vi "SetIntermediateCalibration3.vi"(8 "error in (no error)":errorcluster, 10 "Calibration table":T1={"version"=3, "table type"=60479, "table size"=496, "full version"=67109888, "crc32"=3963612841, "baseline"=-54.831806, "model"=1, "fx left"=917.7658, "fy left"=915.4345, "px left"=631.39185, "py left"=376.6227, "py right"=364.3492, "px right"=651.2822, "fy right"=921.49005, "fx right"=923.5849, "k left"=[0.13533829, -0.40519878, 0.0008784002, -0.0011180333, 0.3588802], "k right"=[0.12740475, -0.39763576, 0.00037952562, -0.0022863527, 0.35284942], "RLeft"=[0.9999986, 0.0009555143, -0.001359244, -0.0009574645, 0.9999985, -0.001434832, 0.001357871, 0.0014361315, 0.99999803], "Rright"=[0.99998456, -0.0019937593, -0.0051888847, 0.002001206, 0.99999696, 0.0014302958, 0.0051860176, -0.0014406577, 0.9999855], "uint8 reserved1"=[0, 0, 0, 0, 0, 0, 0, 0, 0, 0, 0, 0, 0, 0, 0, 0, 0, 0, 0, 0, 0, 0, 0, 0, 0, 0, 0, 0, 0, 0, 0, 0, 0, 0, 0, 0, 0, 0, 0, 0, 0, 0, 0, 0, 0, 0, 0, 0, 0, 0, 0, 0, 0, 0, 0, 0, 0, 0, 0, 0, 0, 0, 0, 0, 0, 0, 0, 0, 0, 0, 0, 0, 0, 0, 0, 0, 0, 0, 0, 0, 0, 0, 0, 0, 0, 0, 0, 0], "uint8 reserved2"=[0, 0, 0, 0, 0, 0, 0, 0, 0, 0, 0, 0, 0, 0, 0, 0, 0, 0, 0, 0, 0, 0, 0, 0, 0, 0, 0, 0, 0, 0, 0, 0, 0, 0, 0, 0, 0, 0, 0, 0, 0, 0, 0, 0, 0, 0, 0, 0, 0, 0, 0, 0, 0, 0, 0, 0, 0, 0, 0, 0, 0, 0, 0, 0], "1920x1080"=[1428.9095, 1428.9095, 951.85925, 556.0496], "1280x720"=[952.6064, 952.6064, 634.5728, 370.69974], "640x480"=[635.0709, 635.0709, 316.38187, 247.13316], "848x480"=[635.0709, 635.0709, 420.38187, 247.13316], "640x360"=[476.3032, 476.3032, 317.2864, 185.34987], "424x240"=[317.53546, 317.53546, 210.19093, 123.56658], "320x240"=[317.53546, 317.53546, 158.19093, 123.56658], "480x270"=[357.2274, 357.2274, 237.96481, 139.0124], "1280x800"=[1058.4515, 1058.4515, 633.9698, 411.8886], "960x540"=[714.4548, 714.4548, 475.92963, 278.0248], "Reserved1"=[714.4548, 714.4548, 475.92963, 278.0248], "Reserved 2"=[714.4548, 714.4548, 475.92963, 278.0248]} {"crc32" format="%x"}, 11 "Input Calibration Parameters":T3={"fx"=0.7094939, "fy"=1.2617997, "px"=0.49358395, "py"=0.4803248, "k left"=[0.13808699, -0.41154006, 0.00043059044, 0.00047021545, 0.34858656], "fx2"=0.7124277, "fy2"=1.2668592, "py2"=0.4684578, "px2"=0.4979801, "k right"=[0.14090613, -0.42654052, -0.0003404384, 0.0005577445, 0.36482877], "RLeft"=[0.99998826, -0.004810224, 0.0006247892, 0.0048055355, 0.9999618, 0.0073000034, -0.00065988, -0.007296915, 0.9999732], "Rright"=[0.9999898, 0.00018351649, -0.0045086313, -0.00021641784, 0.99997336, -0.0072980113, 0.004507172, 0.007298913, 0.9999632], "baseline"=-55.153587, "useBrownModel"=1, "1280x720"=[961.38745, 961.38745, 632.941, 342.07367]}) -> (0 "error out":errorcluster, 2 "size(s)":i32=256, 3 "Intermediate Output":u8[](array[numeric])=[156, 141, 55, 63, 113, 190, 162, 63, 62, 252, 142, 135, 63, 5, 233, 9, 31, 150, 10, 62, 55, 118, 207, 190, 113, 68, 102, 58, 249, 138, 146, 186, 37, 191, 183, 62, 140, 183, 56, 63, 9, 210, 163, 63, 224, 139, 1, 63, 166, 65, 2, 63, 100, 118, 2, 62, 234, 150, 203, 190, 17, 251, 198, 57, 162, 214, 21, 187, 174, 168, 180, 62, 233, 255, 127, 63, 123, 123, 122, 58, 169, 40, 178, 186, 91, 254, 122, 186, 231, 255, 127, 63, 249, 16, 188, 186, 151, 250, 177, 58, 148, 60, 188, 58, 223, 255, 127, 63, 253, 254, 127, 63, 187, 169, 2, 187, 133, 7, 170, 187, 170, 38, 3, 59, 205, 255, 127, 63, 195, 120, 187, 58, 120, 239, 169, 59, 115, 212, 188, 186, 13, 255, 127, 63, 197, 83, 91, 194, 1, 0, 0, 0, 0, 0, 0, 0, 0, 0, 0, 0, 0, 0, 0, 0, 0, 0, 0, 0, 0, 0, 0, 0, 0, 0, 0, 0, 0, 0, 0, 0, 0, 0, 0, 0, 0, 0, 0, 0, 0, 0, 0, 0, 0, 0, 0, 0, 0, 0, 0, 0, 0, 0, 0, 0, 0, 0, 0, 0, 0, 0, 0, 0, 0, 0, 0, 0, 0, 0, 0, 0, 0, 0, 0, 0, 0, 0, 0, 0, 0, 0, 0, 0, 0, 0, 0, 0, 0, 0, 0, 0, 207, 38, 110, 68, 207, 38, 110, 68, 169, 164, 30, 68, 145, 89, 185, 67] format="%x", 4 "New Full cal. output":u8[](array[numeric])=[3, 0, 25, 0, 240, 1, 0, 0, 0, 4, 0, 4, 169, 238, 63, 236, 156, 141, 55, 63, 113, 190, 162, 63, 135, 142, 252, 62, 9, 233, 5, 63, 31, 150, 10, 62, 55, 118, 207, 190, 113, 68, 102, 58, 249, 138, 146, 186, 37, 191, 183, 62, 140, 183, 56, 63, 9, 210, 163, 63, 166, 65, 2, 63, 224, 139, 1, 63, 100, 118, 2, 62, 234, 150, 203, 190, 17, 251, 198, 57, 162, 214, 21, 187, 174, 168, 180, 62, 233, 255, 127, 63, 123, 123, 122, 58, 169, 40, 178, 186, 91, 254, 122, 186, 231, 255, 127, 63, 249, 16, 188, 186, 151, 250, 177, 58, 148, 60, 188, 58, 223, 255, 127, 63, 253, 254, 127, 63, 187, 169, 2, 187, 133, 7, 170, 187, 170, 38, 3, 59, 205, 255, 127, 63, 195, 120, 187, 58, 120, 239, 169, 59, 115, 212, 188, 186, 13, 255, 127, 63, 197, 83, 91, 194, 1, 0, 0, 0, 0, 0, 0, 0, 0, 0, 0, 0, 0, 0, 0, 0, 0, 0, 0, 0, 0, 0, 0, 0, 0, 0, 0, 0, 0, 0, 0, 0, 0, 0, 0, 0, 0, 0, 0, 0, 0, 0, 0, 0, 0, 0, 0, 0, 0, 0, 0, 0, 0, 0, 0, 0, 0, 0, 0, 0, 0, 0, 0, 0, 0, 0, 0, 0, 0, 0, 0, 0, 0, 0, 0, 0, 0, 0, 0, 0, 0, 0, 0, 0, 0, 0, 0, 0, 0, 0, 0, 0, 27, 157, 178, 68, 27, 157, 178, 68, 254, 246, 109, 68, 45, 3, 11, 68, 207, 38, 110, 68, 207, 38, 110, 68, 169, 164, 30, 68, 145, 89, 185, 67, 138, 196, 30, 68, 138, 196, 30, 68, 225, 48, 158, 67, 23, 34, 119, 67, 138, 196, 30, 68, 138, 196, 30, 68, 225, 48, 210, 67, 23, 34, 119, 67, 207, 38, 238, 67, 207, 38, 238, 67, 169, 164, 158, 67, 145, 89, 57, 67, 138, 196, 158, 67, 138, 196, 158, 67, 225, 48, 82, 67, 23, 34, 247, 66, 138, 196, 158, 67, 138, 196, 158, 67, 225, 48, 30, 67, 23, 34, 247, 66, 27, 157, 178, 67, 27, 157, 178, 67, 254, 246, 109, 67, 45, 3, 11, 67, 115, 78, 132, 68, 115, 78, 132, 68, 17, 126, 30, 68, 190, 241, 205, 67, 27, 157, 50, 68, 27, 157, 50, 68, 254, 246, 237, 67, 45, 3, 139, 67, 0, 0, 0, 0, 0, 0, 0, 0, 0, 0, 0, 0, 0, 0, 0, 0, 0, 0, 0, 0, 0, 0, 0, 0, 0, 0, 0, 0, 0, 0, 0, 0, 0, 0, 0, 0, 0, 0, 0, 0, 0, 0, 0, 0, 0, 0, 0, 0, 0, 0, 0, 0, 0, 0, 0, 0, 0, 0, 0, 0, 0, 0, 0, 0, 0, 0, 0, 0, 0, 0, 0, 0, 0, 0, 0, 0, 0, 0, 0, 0, 0, 0, 0, 0, 0, 0, 0, 0, 0, 0, 0, 0, 0, 0, 0, 0] format="%x", 5 "New Calibration table":T1={"version"=3, "table type"=60479, "table size"=496, "full version"=67109888, "crc32"=3963612841, "baseline"=-54.831806, "model"=1, "fx left"=917.7658, "fy left"=915.4345, "px left"=631.39185, "py left"=376.6227, "py right"=364.3492, "px right"=651.2822, "fy right"=921.49005, "fx right"=923.5849, "k left"=[0.13533829, -0.40519878, 0.0008784002, -0.0011180333, 0.3588802], "k right"=[0.12740475, -0.39763576, 0.00037952562, -0.0022863527, 0.35284942], "RLeft"=[0.9999986, 0.0009555143, -0.001359244, -0.0009574645, 0.9999985, -0.001434832, 0.001357871, 0.0014361315, 0.99999803], "Rright"=[0.99998456, -0.0019937593, -0.0051888847, 0.002001206, 0.99999696, 0.0014302958, 0.0051860176, -0.0014406577, 0.9999855], "uint8 reserved1"=[0, 0, 0, 0, 0, 0, 0, 0, 0, 0, 0, 0, 0, 0, 0, 0, 0, 0, 0, 0, 0, 0, 0, 0, 0, 0, 0, 0, 0, 0, 0, 0, 0, 0, 0, 0, 0, 0, 0, 0, 0, 0, 0, 0, 0, 0, 0, 0, 0, 0, 0, 0, 0, 0, 0, 0, 0, 0, 0, 0, 0, 0, 0, 0, 0, 0, 0, 0, 0, 0, 0, 0, 0, 0, 0, 0, 0, 0, 0, 0, 0, 0, 0, 0, 0, 0, 0, 0], "uint8 reserved2"=[0, 0, 0, 0, 0, 0, 0, 0, 0, 0, 0, 0, 0, 0, 0, 0, 0, 0, 0, 0, 0, 0, 0, 0, 0, 0, 0, 0, 0, 0, 0, 0, 0, 0, 0, 0, 0, 0, 0, 0, 0, 0, 0, 0, 0, 0, 0, 0, 0, 0, 0, 0, 0, 0, 0, 0, 0, 0, 0, 0, 0, 0, 0, 0], "1920x1080"=[1428.9095, 1428.9095, 951.85925, 556.0496], "1280x720"=[952.6064, 952.6064, 634.5728, 370.69974], "640x480"=[635.0709, 635.0709, 316.38187, 247.13316], "848x480"=[635.0709, 635.0709, 420.38187, 247.13316], "640x360"=[476.3032, 476.3032, 317.2864, 185.34987], "424x240"=[317.53546, 317.53546, 210.19093, 123.56658], "320x240"=[317.53546, 317.53546, 158.19093, 123.56658], "480x270"=[357.2274, 357.2274, 237.96481, 139.0124], "1280x800"=[1058.4515, 1058.4515, 633.9698, 411.8886], "960x540"=[714.4548, 714.4548, 475.92963, 278.0248], "Reserved1"=[714.4548, 714.4548, 475.92963, 278.0248], "Reserved 2"=[714.4548, 714.4548, 475.92963, 278.0248]} {"crc32" format="%x"}, 6 "New size full":i32=512)   [LabVIEW 2017, in "libRealSense3.lvlib"]
uses:
  libRealSense3.lvlib
panel:
  in  "Calibration table 2":T1={"version"=3, "table type"=60479, "table size"=496, "full version"=67109888, "crc32"=3963612841, "baseline"=-54.831806, "model"=1, "fx left"=917.7658, "fy left"=915.4345, "px left"=631.39185, "py left"=376.6227, "py right"=364.3492, "px right"=651.2822, "fy right"=921.49005, "fx right"=923.5849, "k left"=[0.13533829, -0.40519878, 0.0008784002, -0.0011180333, 0.3588802], "k right"=[0.12740475, -0.39763576, 0.00037952562, -0.0022863527, 0.35284942], "RLeft"=[0.9999986, 0.0009555143, -0.001359244, -0.0009574645, 0.9999985, -0.001434832, 0.001357871, 0.0014361315, 0.99999803], "Rright"=[0.99998456, -0.0019937593, -0.0051888847, 0.002001206, 0.99999696, 0.0014302958, 0.0051860176, -0.0014406577, 0.9999855], "uint8 reserved1"=[0, 0, 0, 0, 0, 0, 0, 0, 0, 0, 0, 0, 0, 0, 0, 0, 0, 0, 0, 0, 0, 0, 0, 0, 0, 0, 0, 0, 0, 0, 0, 0, 0, 0, 0, 0, 0, 0, 0, 0, 0, 0, 0, 0, 0, 0, 0, 0, 0, 0, 0, 0, 0, 0, 0, 0, 0, 0, 0, 0, 0, 0, 0, 0, 0, 0, 0, 0, 0, 0, 0, 0, 0, 0, 0, 0, 0, 0, 0, 0, 0, 0, 0, 0, 0, 0, 0, 0], "uint8 reserved2"=[0, 0, 0, 0, 0, 0, 0, 0, 0, 0, 0, 0, 0, 0, 0, 0, 0, 0, 0, 0, 0, 0, 0, 0, 0, 0, 0, 0, 0, 0, 0, 0, 0, 0, 0, 0, 0, 0, 0, 0, 0, 0, 0, 0, 0, 0, 0, 0, 0, 0, 0, 0, 0, 0, 0, 0, 0, 0, 0, 0, 0, 0, 0, 0], "1920x1080"=[1428.9095, 1428.9095, 951.85925, 556.0496], "1280x720"=[952.6064, 952.6064, 634.5728, 370.69974], "640x480"=[635.0709, 635.0709, 316.38187, 247.13316], "848x480"=[635.0709, 635.0709, 420.38187, 247.13316], "640x360"=[476.3032, 476.3032, 317.2864, 185.34987], "424x240"=[317.53546, 317.53546, 210.19093, 123.56658], "320x240"=[317.53546, 317.53546, 158.19093, 123.56658], "480x270"=[357.2274, 357.2274, 237.96481, 139.0124], "1280x800"=[1058.4515, 1058.4515, 633.9698, 411.8886], "960x540"=[714.4548, 714.4548, 475.92963, 278.0248], "Reserved1"=[714.4548, 714.4548, 475.92963, 278.0248], "Reserved 2"=[714.4548, 714.4548, 475.92963, 278.0248]} {"crc32" format="%x"}
  in  "Tab Control":T2(tab)
  out "Output array":u8[](array[numeric])=[3, 0, 25, 0, 240, 1, 0, 0, 0, 4, 0, 4, 169, 238, 63, 236, 156, 141, 55, 63, 113, 190, 162, 63, 135, 142, 252, 62, 9, 233, 5, 63, 31, 150, 10, 62, 55, 118, 207, 190, 113, 68, 102, 58, 249, 138, 146, 186, 37, 191, 183, 62, 140, 183, 56, 63, 9, 210, 163, 63, 166, 65, 2, 63, 224, 139, 1, 63, 100, 118, 2, 62, 234, 150, 203, 190, 17, 251, 198, 57, 162, 214, 21, 187, 174, 168, 180, 62, 233, 255, 127, 63, 123, 123, 122, 58, 169, 40, 178, 186, 91, 254, 122, 186, 231, 255, 127, 63, 249, 16, 188, 186, 151, 250, 177, 58, 148, 60, 188, 58, 223, 255, 127, 63, 253, 254, 127, 63, 187, 169, 2, 187, 133, 7, 170, 187, 170, 38, 3, 59, 205, 255, 127, 63, 195, 120, 187, 58, 120, 239, 169, 59, 115, 212, 188, 186, 13, 255, 127, 63, 197, 83, 91, 194, 1, 0, 0, 0, 0, 0, 0, 0, 0, 0, 0, 0, 0, 0, 0, 0, 0, 0, 0, 0, 0, 0, 0, 0, 0, 0, 0, 0, 0, 0, 0, 0, 0, 0, 0, 0, 0, 0, 0, 0, 0, 0, 0, 0, 0, 0, 0, 0, 0, 0, 0, 0, 0, 0, 0, 0, 0, 0, 0, 0, 0, 0, 0, 0, 0, 0, 0, 0, 0, 0, 0, 0, 0, 0, 0, 0, 0, 0, 0, 0, 0, 0, 0, 0, 0, 0, 0, 0, 0, 0, 0, 0, 27, 157, 178, 68, 27, 157, 178, 68, 254, 246, 109, 68, 45, 3, 11, 68, 207, 38, 110, 68, 207, 38, 110, 68, 169, 164, 30, 68, 145, 89, 185, 67, 138, 196, 30, 68, 138, 196, 30, 68, 225, 48, 158, 67, 23, 34, 119, 67, 138, 196, 30, 68, 138, 196, 30, 68, 225, 48, 210, 67, 23, 34, 119, 67, 207, 38, 238, 67, 207, 38, 238, 67, 169, 164, 158, 67, 145, 89, 57, 67, 138, 196, 158, 67, 138, 196, 158, 67, 225, 48, 82, 67, 23, 34, 247, 66, 138, 196, 158, 67, 138, 196, 158, 67, 225, 48, 30, 67, 23, 34, 247, 66, 27, 157, 178, 67, 27, 157, 178, 67, 254, 246, 109, 67, 45, 3, 11, 67, 115, 78, 132, 68, 115, 78, 132, 68, 17, 126, 30, 68, 190, 241, 205, 67, 27, 157, 50, 68, 27, 157, 50, 68, 254, 246, 237, 67, 45, 3, 139, 67] format="%x"
  out "Output":i32
  # "RS3 Set Intermediate Calibration 3"
  # "(C) 2018 Intel Corp.,  AGJ"
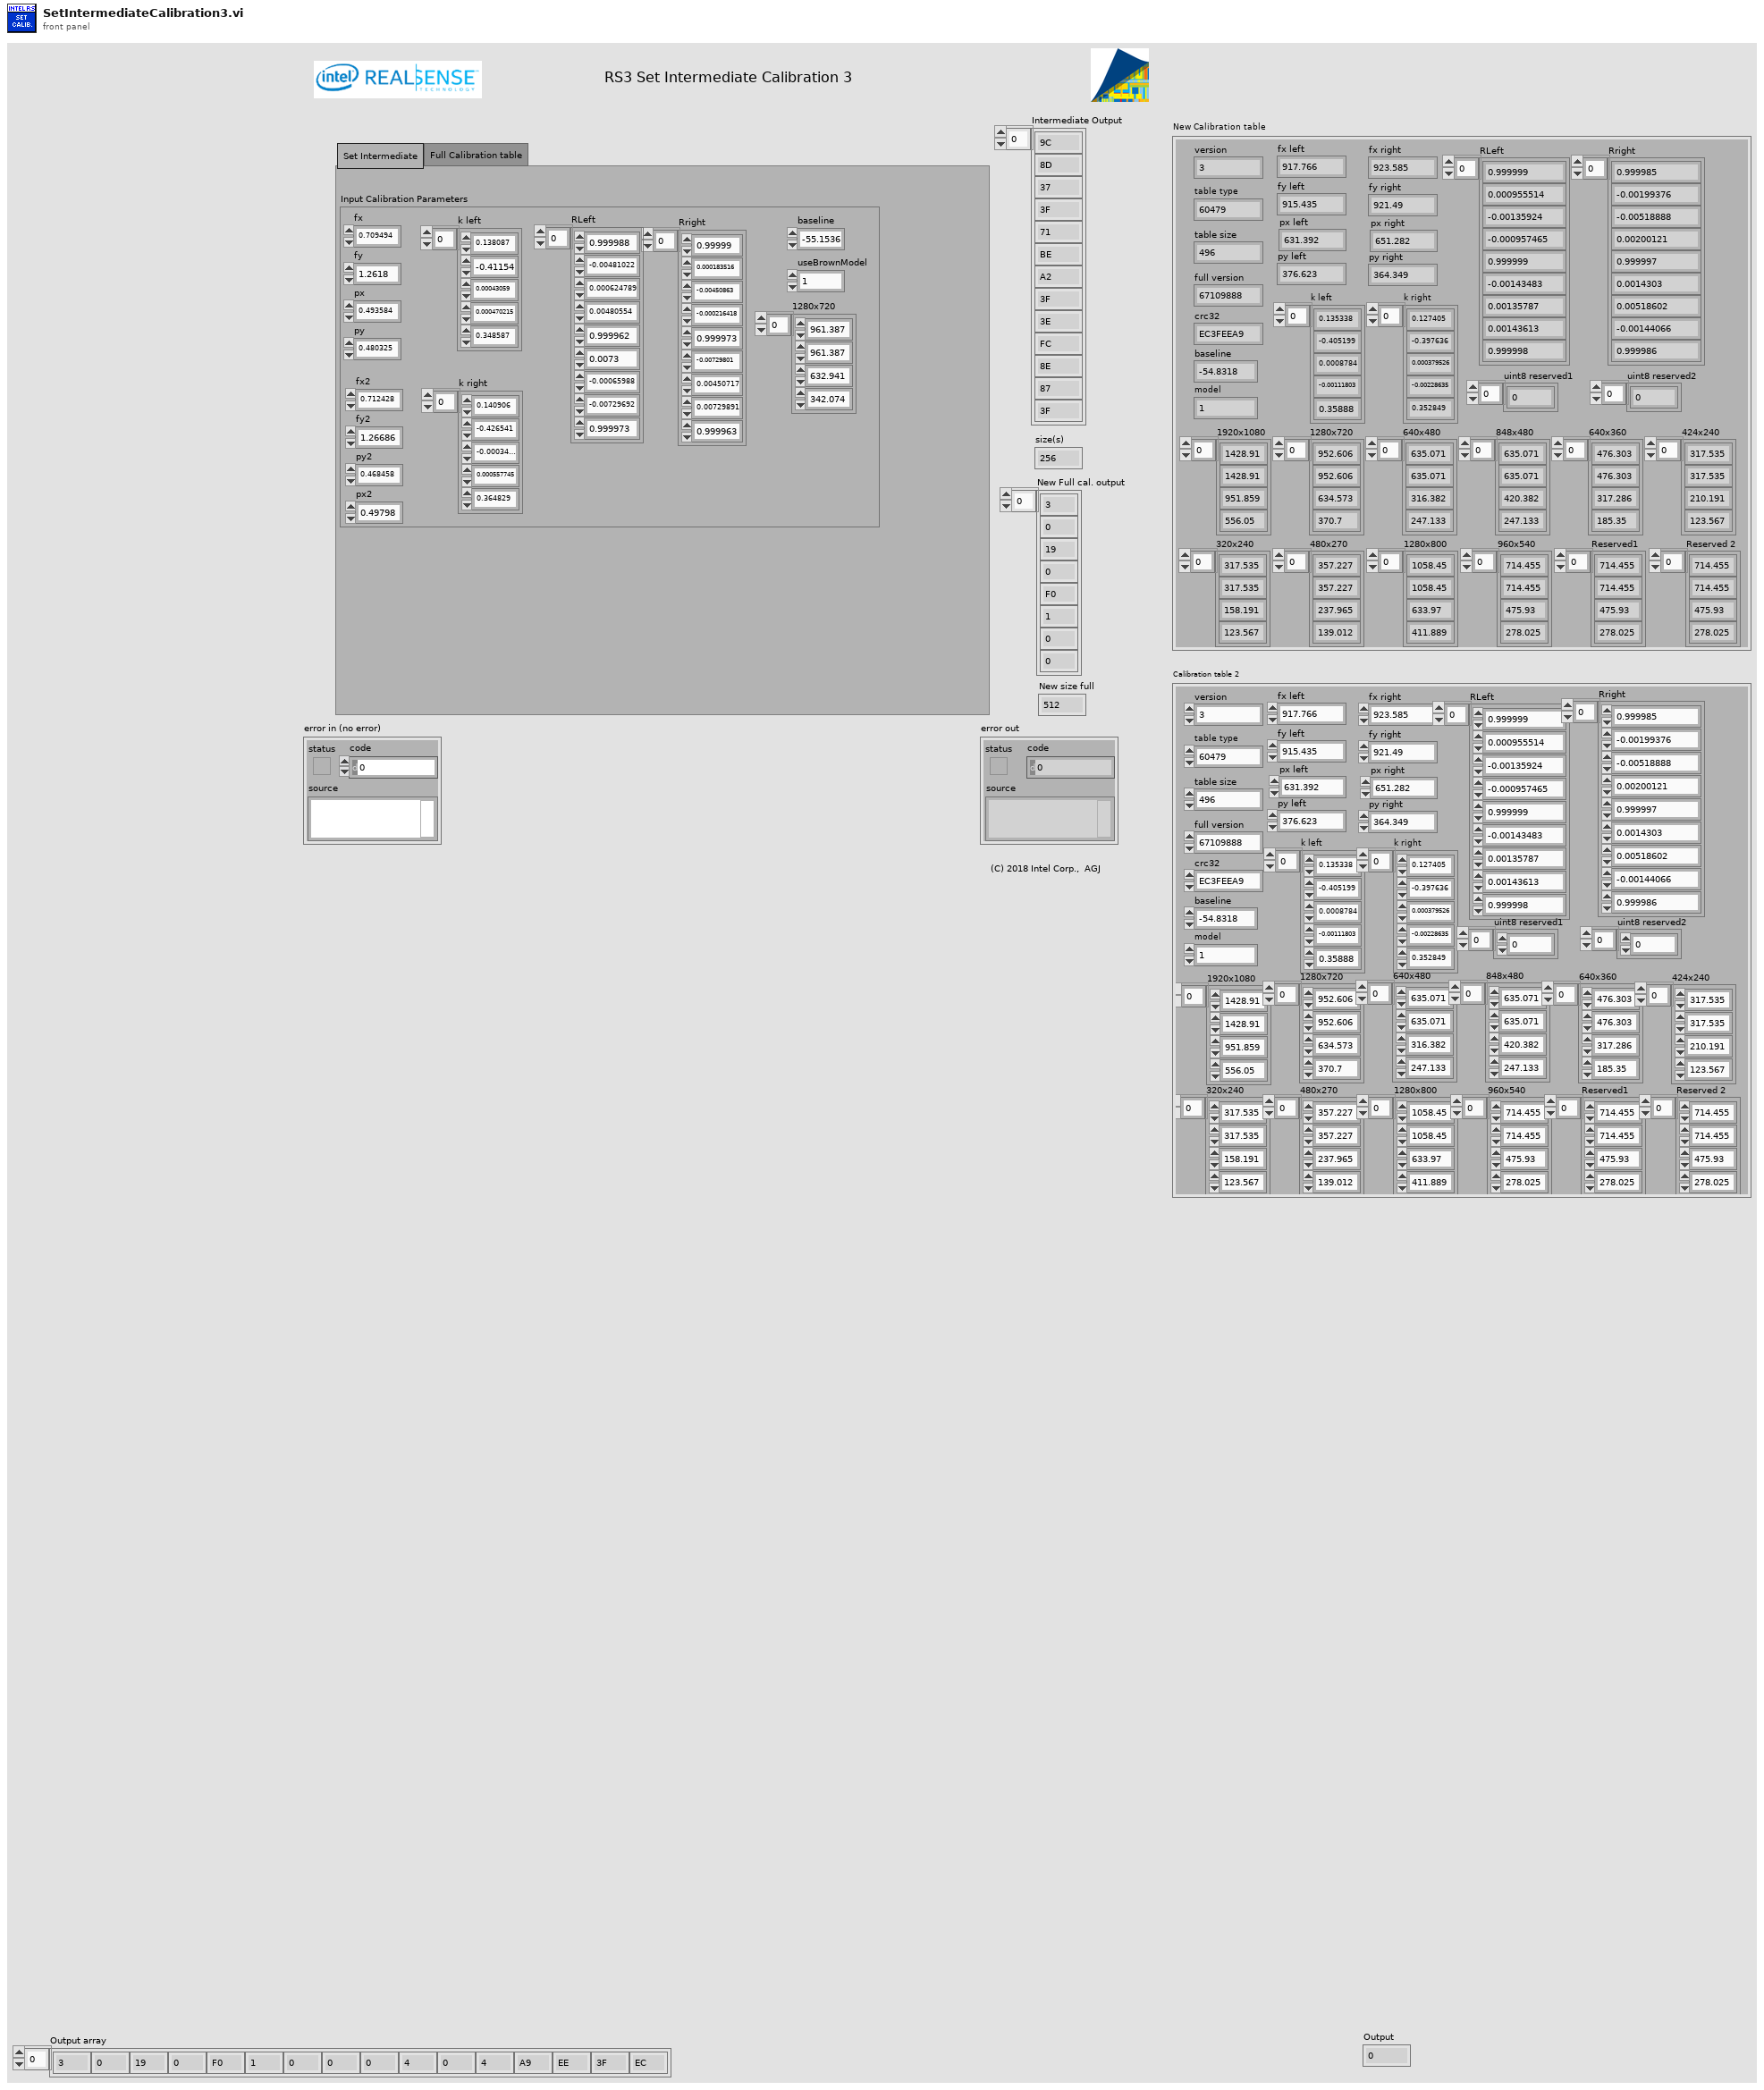
[diagram p1: front panel]
types:
  T1 = cluster{"version":u16, "table type":u16, "table size":u32, "full version":u32, "crc32":u32, "baseline":sgl, "model":u32, "fx left":sgl, "fy left":sgl, "px left":sgl, "py left":sgl, "py right":sgl, "px right":sgl, "fy right":sgl, "fx right":sgl, "k left":sgl[], "k right":sgl[], "RLeft":sgl[], "Rright":sgl[], "uint8 reserved1":u8[], "uint8 reserved2":u8[], "1920x1080":sgl[], "1280x720":sgl[], "640x480":sgl[], "848x480":sgl[], "640x360":sgl[], "424x240":sgl[], "320x240":sgl[], "480x270":sgl[], "1280x800":sgl[], "960x540":sgl[], "Reserved1":sgl[], "Reserved 2":sgl[]}
  T2 = enum32{"Set Intermediate", "Full Calibration table"}
  T3 = cluster{"fx":sgl, "fy":sgl, "px":sgl, "py":sgl, "k left":sgl[], "fx2":sgl, "fy2":sgl, "py2":sgl, "px2":sgl, "k right":sgl[], "RLeft":sgl[], "Rright":sgl[], "baseline":sgl, "useBrownModel":u32, "1280x720":sgl[]}
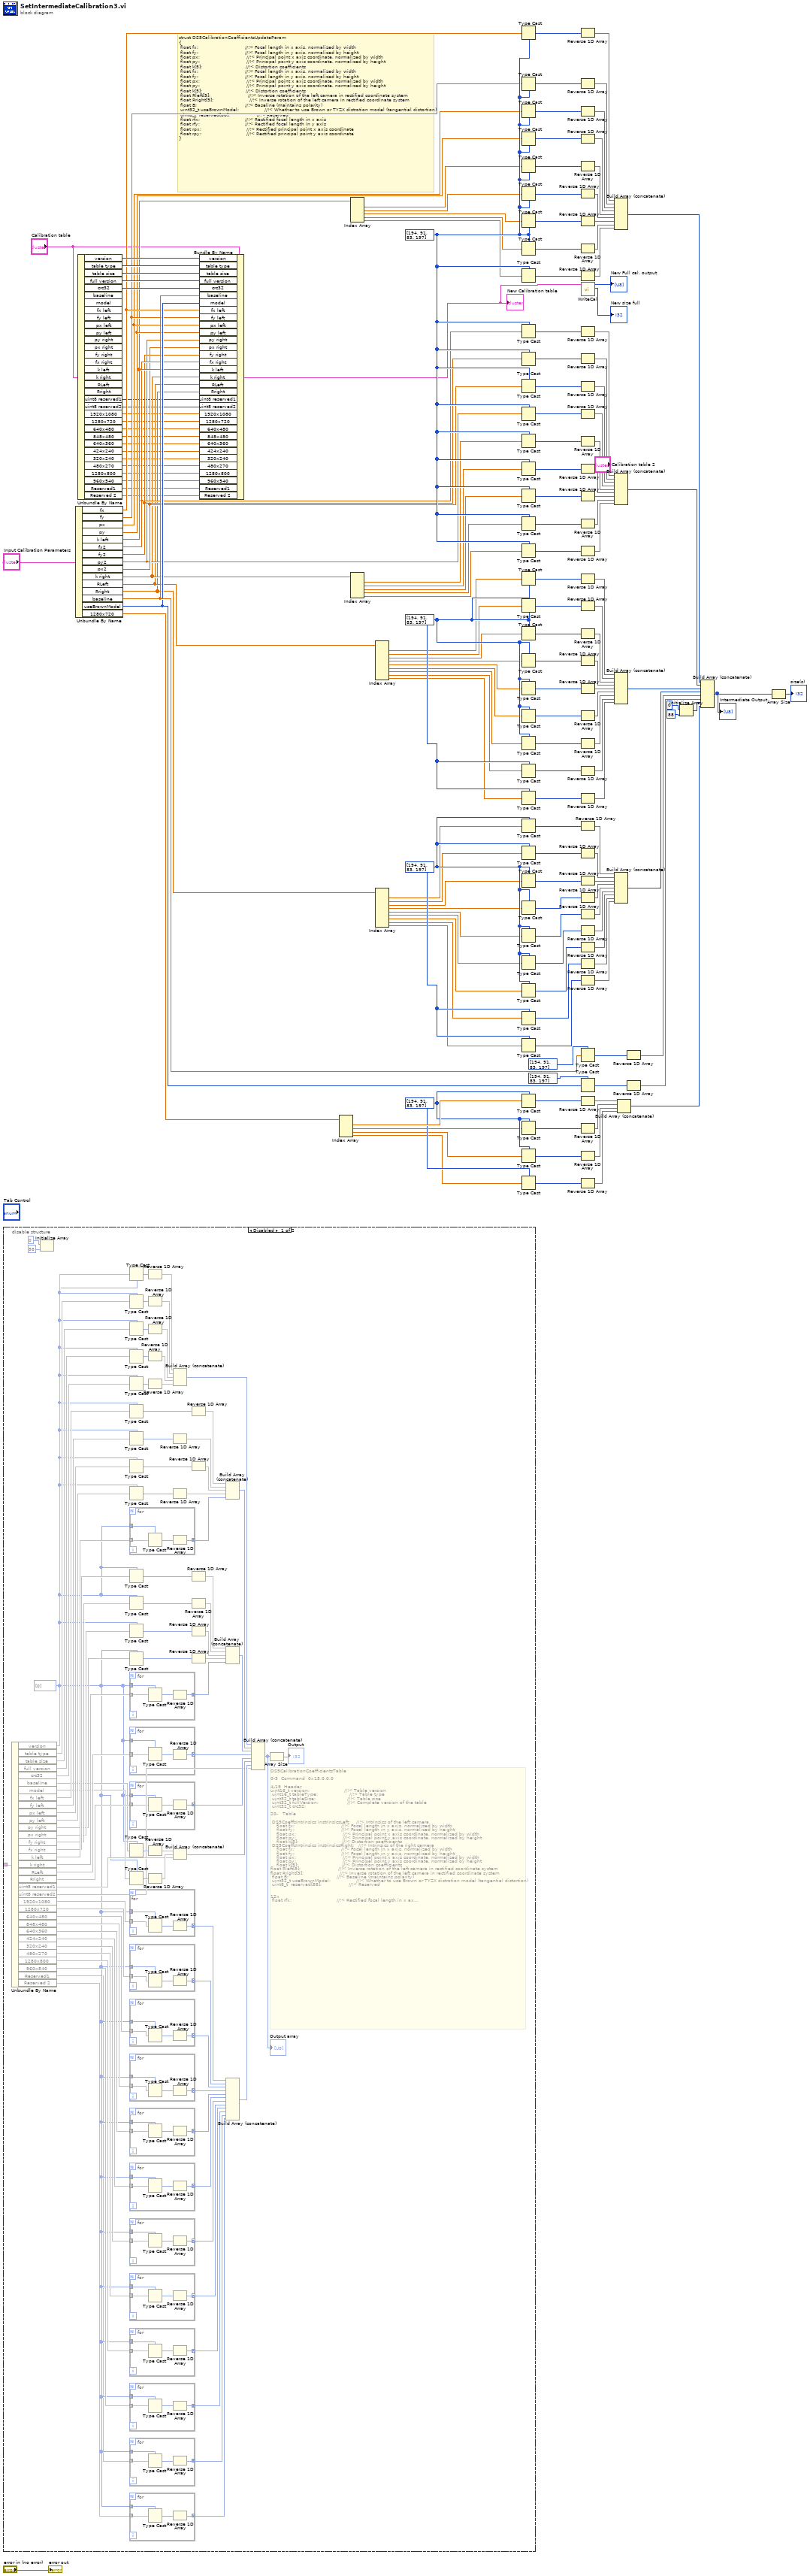
[diagram p0: block diagram]
diagram:
  w56 = u8[] [194, 91, 83, 197] ("reversed array")
  w109 = u8[] [194, 91, 83, 197] ("reversed array")
  w128 = u8[] [194, 91, 83, 197] ("reversed array")
  w147 = u8[] [194, 91, 83, 197] ("reversed array")
  # "struct DS5CalibrationCoefficientsUpdateParam\n{\n\tfloat fx;                               //!< Focal length in x axis, normalized by width\n\tfloat fy;                               //!< Focal length in y axis, normalized by height\n\tfloat px;                               //!< Principal point x axis coordinate, normalized by width\n\tfloat py;                               //!< Principal point y axis coordinate, normalized by height\n\tfloat k[5];                             //!< Distortion coefficients\n\tfloat fx;                               //!< Focal length in x axis, normalized by width\n\tfloat fy;                               //!< Focal length in y axis, normalized by height\n\tfloat px;                               //!< Principal point x axis coordinate, normalized by width\n\tfloat py;                               //!< Principal point y axis coordinate, normalized by height\n\tfloat k[5];                             //!< Distortion coefficients\n\tfloat Rleft[9];                         //!< Inverse rotation of the left camera in rectified coordinate system\n\tfloat Rright[9];                        //!< Inverse rotation of the left camera in rectified coordinate system\n\tfloat B;                                //!< Baseline (maintains polarity)\n\tuint32_t useBrownModel;                 //!< Whether to use Brown or TYZX distrotion model (tangential distortion)\n\tuint8_t  reserved[88];                  //!< Reserved\n\tfloat rfx;                              //!< Rectified focal length in x axis\n\tfloat rfy;                              //!< Rectified focal length in y axis\n\tfloat rpx;                              //!< Rectified principal point x axis coordinate\n\tfloat rpy;                              //!< Rectified principal point y axis coordinate\n}"
  n1 = disable-structure shown="Disabled" {
    disable-tunnel: _ -> [w262 _]
    frame Disabled {
      w178 = u8[] [0]
      # "DS5CalibrationCoefficientsTable\n\n0-3  Command  0x15,0,0,0\n\n4-19\t Header\nuint16_t version;                       //!< Table version\n\tuint16_t tableType;                     //!< Table type\n\tuint32_t tableSize;                     //!< Table size \n\tuint32_t fullVersion;                   //!< Complete version of the table\n\tuint32_t crc32; \n\n20-   Table\n\n\tDS5CoeffsIntrinsics instrinsicsLeft;    //!< Intrinsics of the left camera\n   \tfloat fx;                               //!< Focal length in x axis, normalized by width\n   \tfloat fy;                               //!< Focal length in y axis, normalized by height\n\t   float px;                               //!< Principal point x axis coordinate, normalized by width\n\t   float py;                               //!< Principal point y axis coordinate, normalized by height\n\t   float k[5];                             //!< Distortion coefficients\n\tDS5CoeffsIntrinsics instrinsicsRight;   //!< Intrinsics of the right camera\n   \tfloat fx;                               //!< Focal length in x axis, normalized by width\n   \tfloat fy;                               //!< Focal length in y axis, normalized by height\n\t   float px;                               //!< Principal point x axis coordinate, normalized by width\n\t   float py;                               //!< Principal point y axis coordinate, normalized by height\n\t   float k[5];                             //!< Distortion coefficients\t\nfloat Rleft[9];                         //!< Inverse rotation of the left camera in rectified coordinate system\nfloat Rright[9];                        //!< Inverse rotation of the left camera in rectified coordinate system\n\tfloat B;                                //!< Baseline (maintains polarity)\n\tuint32_t useBrownModel;                 //!< Whether to use Brown or TYZX distrotion model (tangential distortion)\n\tuint8_t  reserved[88];                  //!< Reserved\n\n\n12x \n\tfloat rfx;                              //!< Rectified focal length in x axis\n\tfloat rfy;                              //!< Rectified focal length in y axis\n\tfloat rpx;                              //!< Rectified principal point x axis coordinate\n\tfloat rpy;                              //!< Rectified principal point y axis coordinate\n\n64x reserved"
      n2 = Unbundle By Name(w262) -> ("version"=w260, "table type"=w258, "table size"=w256, "full version"=w251, "crc32"=w249, "baseline"=w210, "model"=w208, "fx left"=w245, "fy left"=w243, "px left"=w242, "py left"=w241, "py right"=w218, "px right"=w219, "fy right"=w220, "fx right"=w221, "k left"=w231, "k right"=w217, "RLeft"=w215, "Rright"=w214, "uint8 reserved1"=w201, "uint8 reserved2"=w179, "1920x1080"=w202, "1280x720"=w200, "640x480"=w199, "848x480"=w198, "640x360"=w197, "424x240"=w196, "320x240"=w195, "480x270"=w194, "1280x800"=w193, "960x540"=w192, "Reserved1"=w174, "Reserved 2"=w173)
      n3 = Initialize Array(u8 0 ("element"), 88 ("dimension size")) -> ()  [unwired: 1 out]
      n4 = Type Cast(type=w178, x=w260) -> (*(type *) &x=w261:u8[])
      n5 = Type Cast(type=w178, x=w258) -> (*(type *) &x=w259:u8[])
      n6 = Type Cast(type=w178, x=w256) -> (*(type *) &x=w257:u8[])
      n7 = Type Cast(type=w178, x=w251) -> (*(type *) &x=w252:u8[])
      n8 = Type Cast(type=w178, x=w249) -> (*(type *) &x=w248:u8[])
      n9 = Type Cast(type=w178, x=w245) -> (*(type *) &x=w246:u8[])
      n10 = Type Cast(type=w178, x=w243) -> (*(type *) &x=w240:u8[])
      n11 = Type Cast(type=w178, x=w242) -> (*(type *) &x=w239:u8[])
      n12 = Type Cast(type=w178, x=w241) -> (*(type *) &x=w238:u8[])
      n13 = for {
        tunnel: [w325] -> w232 mode=concatenating
        tunnel: w231 -> [w324]
        tunnel: w178 -> [w323]
        n14 = Type Cast(type=w323, x=w324) -> (*(type *) &x=w326:u8[])
        n15 = Reverse 1D Array(array=w326) -> (reversed array=w325:u8[])
      }
      n16 = Type Cast(type=w178, x=w221) -> (*(type *) &x=w222:u8[])
      n17 = Type Cast(type=w178, x=w220) -> (*(type *) &x=w224:u8[])
      n18 = Type Cast(type=w178, x=w219) -> (*(type *) &x=w225:u8[])
      n19 = Type Cast(type=w178, x=w218) -> (*(type *) &x=w226:u8[])
      n20 = for {
        tunnel: [w321] -> w230 mode=concatenating
        tunnel: w178 -> [w320]
        tunnel: w217 -> [w319]
        n21 = Type Cast(type=w320, x=w319) -> (*(type *) &x=w322:u8[])
        n22 = Reverse 1D Array(array=w322) -> (reversed array=w321:u8[])
      }
      n23 = for {
        tunnel: [w317] -> w213 mode=concatenating
        tunnel: w178 -> [w316]
        tunnel: w215 -> [w315]
        n24 = Type Cast(type=w316, x=w315) -> (*(type *) &x=w318:u8[])
        n25 = Reverse 1D Array(array=w318) -> (reversed array=w317:u8[])
      }
      n26 = for {
        tunnel: [w313] -> w212 mode=concatenating
        tunnel: w178 -> [w312]
        tunnel: w214 -> [w311]
        n27 = Type Cast(type=w312, x=w311) -> (*(type *) &x=w314:u8[])
        n28 = Reverse 1D Array(array=w314) -> (reversed array=w313:u8[])
      }
      n29 = Type Cast(type=w178, x=w210) -> (*(type *) &x=w211:u8[])
      n30 = Type Cast(type=w178, x=w208) -> (*(type *) &x=w209:u8[])
      n31 = for {
        tunnel: [w309] -> w191 mode=concatenating
        tunnel: w178 -> [w308]
        tunnel: w202 -> [w307]
        n32 = Type Cast(type=w308, x=w307) -> (*(type *) &x=w310:u8[])
        n33 = Reverse 1D Array(array=w310) -> (reversed array=w309:u8[])
      }
      n34 = for {
        tunnel: [w305] -> w190 mode=concatenating
        tunnel: w178 -> [w304]
        tunnel: w200 -> [w303]
        n35 = Type Cast(type=w304, x=w303) -> (*(type *) &x=w306:u8[])
        n36 = Reverse 1D Array(array=w306) -> (reversed array=w305:u8[])
      }
      n37 = for {
        tunnel: [w301] -> w189 mode=concatenating
        tunnel: w178 -> [w300]
        tunnel: w199 -> [w299]
        n38 = Type Cast(type=w300, x=w299) -> (*(type *) &x=w302:u8[])
        n39 = Reverse 1D Array(array=w302) -> (reversed array=w301:u8[])
      }
      n40 = for {
        tunnel: [w297] -> w188 mode=concatenating
        tunnel: w178 -> [w296]
        tunnel: w198 -> [w295]
        n41 = Type Cast(type=w296, x=w295) -> (*(type *) &x=w298:u8[])
        n42 = Reverse 1D Array(array=w298) -> (reversed array=w297:u8[])
      }
      n43 = for {
        tunnel: [w293] -> w187 mode=concatenating
        tunnel: w178 -> [w292]
        tunnel: w197 -> [w291]
        n44 = Type Cast(type=w292, x=w291) -> (*(type *) &x=w294:u8[])
        n45 = Reverse 1D Array(array=w294) -> (reversed array=w293:u8[])
      }
      n46 = for {
        tunnel: [w289] -> w186 mode=concatenating
        tunnel: w178 -> [w288]
        tunnel: w196 -> [w287]
        n47 = Type Cast(type=w288, x=w287) -> (*(type *) &x=w290:u8[])
        n48 = Reverse 1D Array(array=w290) -> (reversed array=w289:u8[])
      }
      n49 = for {
        tunnel: [w285] -> w185 mode=concatenating
        tunnel: w178 -> [w284]
        tunnel: w195 -> [w283]
        n50 = Type Cast(type=w284, x=w283) -> (*(type *) &x=w286:u8[])
        n51 = Reverse 1D Array(array=w286) -> (reversed array=w285:u8[])
      }
      n52 = for {
        tunnel: [w281] -> w184 mode=concatenating
        tunnel: w178 -> [w280]
        tunnel: w194 -> [w279]
        n53 = Type Cast(type=w280, x=w279) -> (*(type *) &x=w282:u8[])
        n54 = Reverse 1D Array(array=w282) -> (reversed array=w281:u8[])
      }
      n55 = for {
        tunnel: [w277] -> w183 mode=concatenating
        tunnel: w178 -> [w276]
        tunnel: w193 -> [w275]
        n56 = Type Cast(type=w276, x=w275) -> (*(type *) &x=w278:u8[])
        n57 = Reverse 1D Array(array=w278) -> (reversed array=w277:u8[])
      }
      n58 = for {
        tunnel: [w273] -> w182 mode=concatenating
        tunnel: w178 -> [w272]
        tunnel: w192 -> [w271]
        n59 = Type Cast(type=w272, x=w271) -> (*(type *) &x=w274:u8[])
        n60 = Reverse 1D Array(array=w274) -> (reversed array=w273:u8[])
      }
      n61 = for {
        tunnel: [w269] -> w177 mode=concatenating
        tunnel: w178 -> [w268]
        tunnel: w174 -> [w267]
        n62 = Type Cast(type=w268, x=w267) -> (*(type *) &x=w270:u8[])
        n63 = Reverse 1D Array(array=w270) -> (reversed array=w269:u8[])
      }
      n64 = for {
        tunnel: [w265] -> w176 mode=concatenating
        tunnel: w178 -> [w264]
        tunnel: w173 -> [w263]
        n65 = Type Cast(type=w264, x=w263) -> (*(type *) &x=w266:u8[])
        n66 = Reverse 1D Array(array=w266) -> (reversed array=w265:u8[])
      }
      n67 = Reverse 1D Array(array=w261) -> (reversed array=w255:u8[])
      n68 = Reverse 1D Array(array=w259) -> (reversed array=w254:u8[])
      n69 = Reverse 1D Array(array=w257) -> (reversed array=w253:u8[])
      n70 = Reverse 1D Array(array=w252) -> (reversed array=w250:u8[])
      n71 = Reverse 1D Array(array=w248) -> (reversed array=w247:u8[])
      n72 = Reverse 1D Array(array=w211) -> (reversed array=w206:u8[])
      n73 = Reverse 1D Array(array=w209) -> (reversed array=w205:u8[])
      n74 = Build Array (concatenate)(w255, w254, w253, w250, w247) -> (w234:u8[])
      n75 = Reverse 1D Array(array=w240) -> (reversed array=w237:u8[])
      n76 = Reverse 1D Array(array=w238) -> (reversed array=w235:u8[])
      n77 = Build Array (concatenate)(w206, w205, w201) -> (w204:u8[])
      n78 = Reverse 1D Array(array=w246) -> (reversed array=w244:u8[])
      n79 = Reverse 1D Array(array=w239) -> (reversed array=w236:u8[])
      n80 = Reverse 1D Array(array=w222) -> (reversed array=w223:u8[])
      n81 = Reverse 1D Array(array=w224) -> (reversed array=w227:u8[])
      n82 = Reverse 1D Array(array=w225) -> (reversed array=w228:u8[])
      n83 = Reverse 1D Array(array=w226) -> (reversed array=w229:u8[])
      n84 = Build Array (concatenate)(w244, w237, w236, w235, w232) -> (w233:u8[])
      n85 = Build Array (concatenate)(w223, w227, w228, w229, w230) -> (w216:u8[])
      n86 = Build Array (concatenate)(w191, w190, w189, w188, w187, w186, w185, w184, w183, w182, w177, w176) -> (w181:u8[])
      n87 = Build Array (concatenate)(w234, w233, w216, w213, w212, w204, w181, w179) -> (w175:u8[])
      "Output array" <- w175
      n88 = Array Size(array=w175) -> (size(s)=→"Output":i32)
    }
    frame Enabled {
    }
  }
  n89 = Unbundle By Name("Input Calibration Parameters") -> ("fx"=w31:sgl, "fy"=w30:sgl, "px"=w29:sgl, "py"=w28:sgl, "k left"=w27:sgl[], "fx2"=w26:sgl, "fy2"=w25:sgl, "py2"=w23:sgl, "px2"=w24:sgl, "k right"=w22:sgl[], "RLeft"=w21:sgl[], "Rright"=w20:sgl[], "baseline"=w33:sgl, "useBrownModel"=w32:u32, "1280x720"=w17:sgl[])
  n90 = Unbundle By Name("Calibration table") -> ("version"=w38:u16, "table type"=w37:u16, "table size"=w36:u32, "full version"=w35:u32, "crc32"=w34:u32, "uint8 reserved1"=w19:u8[], "uint8 reserved2"=w18:u8[], "1920x1080"=w16:sgl[], "1280x720"=w1:sgl[], "640x480"=w15:sgl[], "848x480"=w14:sgl[], "640x360"=w13:sgl[], "424x240"=w12:sgl[], "320x240"=w11:sgl[], "480x270"=w10:sgl[], "1280x800"=w9:sgl[], "960x540"=w8:sgl[], "Reserved1"=w7:sgl[], "Reserved 2"=w6:sgl[])  [unwired: 14 out]
  n91 = Bundle By Name(cluster="Calibration table", "version"=w38, "table type"=w37, "table size"=w36, "full version"=w35, "crc32"=w34, "baseline"=w33, "model"=w32, "fx left"=w31, "fy left"=w30, "px left"=w29, "py left"=w28, "py right"=w23, "px right"=w24, "fy right"=w25, "fx right"=w26, "k left"=w27, "k right"=w22, "RLeft"=w21, "Rright"=w20, "uint8 reserved1"=w19, "uint8 reserved2"=w18, "1920x1080"=w16, "1280x720"=w1, "640x480"=w15, "848x480"=w14, "640x360"=w13, "424x240"=w12, "320x240"=w11, "480x270"=w10, "1280x800"=w9, "960x540"=w8, "Reserved1"=w7, "Reserved 2"=w6) -> (w2:T1)
  "New Calibration table" <- w2
  n92 = Index Array(array=w17) -> (element #1=w57:sgl, element #2=w55:sgl, element #3=w54:sgl, element #4=w53:sgl)  [unwired: 4 in]
  n93 = Index Array(array=w27) -> (element #1=w79:sgl, element #2=w78:sgl, element #3=w77:sgl, element #4=w76:sgl, element #5=w75:sgl)  [unwired: 5 in]
  n94 = Index Array(array=w22) -> (element #1=w74:sgl, element #2=w73:sgl, element #3=w72:sgl, element #4=w71:sgl, element #5=w70:sgl)  [unwired: 5 in]
  n95 = Index Array(array=w21) -> (element #1=w97:sgl, element #2=w96:sgl, element #3=w95:sgl, element #4=w94:sgl, element #5=w93:sgl, element #6=w92:sgl, element #7=w91:sgl, element #8=w90:sgl, element #9=w89:sgl)  [unwired: 9 in]
  n96 = Index Array(array=w20) -> (element #1=w88:sgl, element #2=w87:sgl, element #3=w86:sgl, element #4=w85:sgl, element #5=w84:sgl, element #6=w83:sgl, element #7=w82:sgl, element #8=w81:sgl, element #9=w80:sgl)  [unwired: 9 in]
  n97 = Type Cast(type=w147, x=w31) -> (*(type *) &x=w172:u8[])
  n98 = Type Cast(type=w147, x=w30) -> (*(type *) &x=w171:u8[])
  n99 = Type Cast(type=w147, x=w29) -> (*(type *) &x=w168:u8[])
  n100 = Type Cast(type=w147, x=w28) -> (*(type *) &x=w167:u8[])
  n101 = Type Cast(type=w147, x=w79) -> (*(type *) &x=w162:u8[])
  n102 = Type Cast(type=w147, x=w78) -> (*(type *) &x=w161:u8[])
  n103 = Type Cast(type=w147, x=w77) -> (*(type *) &x=w160:u8[])
  n104 = Type Cast(type=w147, x=w76) -> (*(type *) &x=w159:u8[])
  n105 = Type Cast(type=w147, x=w75) -> (*(type *) &x=w154:u8[])
  n106 = Type Cast(type=w147, x=w26) -> (*(type *) &x=w163:u8[])
  n107 = Type Cast(type=w147, x=w25) -> (*(type *) &x=w164:u8[])
  n108 = Type Cast(type=w147, x=w24) -> (*(type *) &x=w165:u8[])
  n109 = Type Cast(type=w147, x=w23) -> (*(type *) &x=w166:u8[])
  n110 = Type Cast(type=w147, x=w74) -> (*(type *) &x=w152:u8[])
  n111 = Type Cast(type=w147, x=w73) -> (*(type *) &x=w151:u8[])
  n112 = Type Cast(type=w147, x=w72) -> (*(type *) &x=w150:u8[])
  n113 = Type Cast(type=w147, x=w71) -> (*(type *) &x=w149:u8[])
  n114 = Type Cast(type=w147, x=w70) -> (*(type *) &x=w148:u8[])
  n115 = Type Cast(type=w128, x=w97) -> (*(type *) &x=w137:u8[])
  n116 = Type Cast(type=w128, x=w96) -> (*(type *) &x=w136:u8[])
  n117 = Type Cast(type=w128, x=w95) -> (*(type *) &x=w135:u8[])
  n118 = Type Cast(type=w128, x=w94) -> (*(type *) &x=w134:u8[])
  n119 = Type Cast(type=w128, x=w93) -> (*(type *) &x=w133:u8[])
  n120 = Type Cast(type=w128, x=w92) -> (*(type *) &x=w132:u8[])
  n121 = Type Cast(type=w128, x=w91) -> (*(type *) &x=w131:u8[])
  n122 = Type Cast(type=w128, x=w90) -> (*(type *) &x=w130:u8[])
  n123 = Type Cast(type=w128, x=w89) -> (*(type *) &x=w129:u8[])
  n124 = Type Cast(type=w109, x=w88) -> (*(type *) &x=w100:u8[])
  n125 = Type Cast(type=w109, x=w87) -> (*(type *) &x=w101:u8[])
  n126 = Type Cast(type=w109, x=w86) -> (*(type *) &x=w102:u8[])
  n127 = Type Cast(type=w109, x=w85) -> (*(type *) &x=w103:u8[])
  n128 = Type Cast(type=w109, x=w84) -> (*(type *) &x=w104:u8[])
  n129 = Type Cast(type=w109, x=w83) -> (*(type *) &x=w105:u8[])
  n130 = Type Cast(type=w109, x=w82) -> (*(type *) &x=w106:u8[])
  n131 = Type Cast(type=w109, x=w81) -> (*(type *) &x=w107:u8[])
  n132 = Type Cast(type=w109, x=w80) -> (*(type *) &x=w108:u8[])
  n133 = Type Cast(type=w56, x=w57) -> (*(type *) &x=w58:u8[])
  n134 = Type Cast(type=w56, x=w55) -> (*(type *) &x=w50:u8[])
  n135 = Type Cast(type=w56, x=w54) -> (*(type *) &x=w51:u8[])
  n136 = Type Cast(type=w56, x=w53) -> (*(type *) &x=w52:u8[])
  n137 = Reverse 1D Array(array=w172) -> (reversed array=w170:u8[])
  n138 = Reverse 1D Array(array=w171) -> (reversed array=w169:u8[])
  n139 = Reverse 1D Array(array=w168) -> (reversed array=w40:u8[])
  n140 = Reverse 1D Array(array=w167) -> (reversed array=w39:u8[])
  n141 = Reverse 1D Array(array=w162) -> (reversed array=w158:u8[])
  n142 = Reverse 1D Array(array=w161) -> (reversed array=w157:u8[])
  n143 = Reverse 1D Array(array=w160) -> (reversed array=w156:u8[])
  n144 = Reverse 1D Array(array=w159) -> (reversed array=w155:u8[])
  n145 = Reverse 1D Array(array=w154) -> (reversed array=w153:u8[])
  n146 = call "WriteCal.vi"("Calibration table"=w2) -> ("size"=→"New size full":i32, "Output array"=→"New Full cal. output":u8[])  [unwired: 9 in]
  n147 = Reverse 1D Array(array=w163) -> (reversed array=w146:u8[])
  n148 = Reverse 1D Array(array=w164) -> (reversed array=w145:u8[])
  n149 = Reverse 1D Array(array=w165) -> (reversed array=w144:u8[])
  n150 = Reverse 1D Array(array=w166) -> (reversed array=w143:u8[])
  n151 = Reverse 1D Array(array=w152) -> (reversed array=w142:u8[])
  n152 = Reverse 1D Array(array=w151) -> (reversed array=w141:u8[])
  n153 = Reverse 1D Array(array=w150) -> (reversed array=w140:u8[])
  n154 = Reverse 1D Array(array=w149) -> (reversed array=w139:u8[])
  n155 = Reverse 1D Array(array=w148) -> (reversed array=w138:u8[])
  n156 = Reverse 1D Array(array=w137) -> (reversed array=w127:u8[])
  n157 = Reverse 1D Array(array=w136) -> (reversed array=w126:u8[])
  n158 = Reverse 1D Array(array=w135) -> (reversed array=w125:u8[])
  n159 = Reverse 1D Array(array=w134) -> (reversed array=w124:u8[])
  n160 = Reverse 1D Array(array=w133) -> (reversed array=w123:u8[])
  n161 = Reverse 1D Array(array=w132) -> (reversed array=w122:u8[])
  n162 = Reverse 1D Array(array=w131) -> (reversed array=w121:u8[])
  n163 = Reverse 1D Array(array=w130) -> (reversed array=w120:u8[])
  n164 = Reverse 1D Array(array=w129) -> (reversed array=w119:u8[])
  n165 = Reverse 1D Array(array=w100) -> (reversed array=w110:u8[])
  n166 = Reverse 1D Array(array=w101) -> (reversed array=w111:u8[])
  n167 = Reverse 1D Array(array=w102) -> (reversed array=w112:u8[])
  n168 = Reverse 1D Array(array=w103) -> (reversed array=w113:u8[])
  n169 = Reverse 1D Array(array=w104) -> (reversed array=w114:u8[])
  n170 = Reverse 1D Array(array=w105) -> (reversed array=w115:u8[])
  n171 = Reverse 1D Array(array=w106) -> (reversed array=w116:u8[])
  n172 = Reverse 1D Array(array=w107) -> (reversed array=w117:u8[])
  n173 = Reverse 1D Array(array=w108) -> (reversed array=w118:u8[])
  n174 = Type Cast(type=u8[] [194, 91, 83, 197] ("reversed array"), x=w33) -> (*(type *) &x=w99:u8[])
  n175 = Type Cast(type=u8[] [194, 91, 83, 197] ("reversed array"), x=w32) -> (*(type *) &x=w68:u8[])
  n176 = Reverse 1D Array(array=w58) -> (reversed array=w49:u8[])
  n177 = Reverse 1D Array(array=w50) -> (reversed array=w48:u8[])
  n178 = Reverse 1D Array(array=w51) -> (reversed array=w47:u8[])
  n179 = Reverse 1D Array(array=w52) -> (reversed array=w46:u8[])
  n180 = Build Array (concatenate)(w170, w169, w40, w39, w158, w157, w156, w155, w153) -> (w65:u8[])
  n181 = Build Array (concatenate)(w146, w145, w144, w143, w142, w141, w140, w139, w138) -> (w64:u8[])
  n182 = Build Array (concatenate)(w127, w126, w125, w124, w123, w122, w121, w120, w119) -> (w63:u8[])
  n183 = Build Array (concatenate)(w110, w111, w112, w113, w114, w115, w116, w117, w118) -> (w62:u8[])
  n184 = Build Array (concatenate)(w49, w48, w47, w46) -> (w45:u8[])
  n185 = Reverse 1D Array(array=w99) -> (reversed array=w61:u8[])
  n186 = Reverse 1D Array(array=w68) -> (reversed array=w60:u8[])
  n187 = Initialize Array(u8 0, 88 ("dimension size")) -> (w59:u8[])
  n188 = Build Array (concatenate)(w65, w64, w63, w62, w61, w60, w59, w45) -> (w44:u8[])
  "Intermediate Output" <- w44
  n189 = Array Size(array=w44) -> (size(s)=→"size(s)":i32)
  "error out" <- "error in (no error)"
